vi "ql2proto_message_compose.vi"(10 "query":string, 11 "token":u64 format="%016x") -> (3 "tcp_write":string)   [LabVIEW 2017]
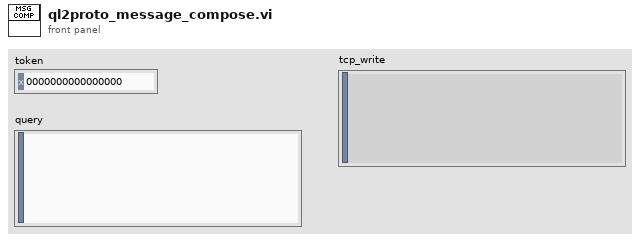
[diagram p1: front panel]
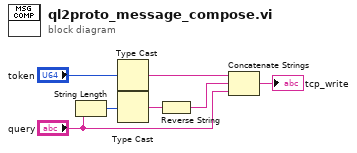
[diagram p0: block diagram]
diagram:
  n1 = String Length(string="query") -> (length=w6:i32)
  n2 = Type Cast(x="token") -> (*(type *) &x=w4:string)  [unwired: 1 in]
  n3 = Type Cast(x=w6) -> (*(type *) &x=w5:string)  [unwired: 1 in]
  n4 = Reverse String(1:w5) -> (0:w3:string)
  n5 = Concatenate Strings(w4, w3, "query") -> (→"tcp_write":string)
